vi "Simple Client - Front Panel.vi"() -> ()   [LabVIEW 2011]
uses:
  <vilib>/variable/tagger/epics/API/internal/List Records (By Ref).vi
  <vilib>/variable/tagger/epics/API/NI_EPICS_Client.lvlib
  <vilib>/lvdsc/NI_DSC.lvlib
  Program Files (x86)/National Instruments/LabVIEW 2011/resource/objmgr/nvio.rc
panel:
  in  "Host":string="localhost" caption="IOC Host"
  in  "Process Variable":string caption="Process Variable to Read (Numeric Only)"
  in  "Exit":bool
  out "Value History":dbl(graph)
  out "Value":dbl(knob) scale=-100.0..100.0
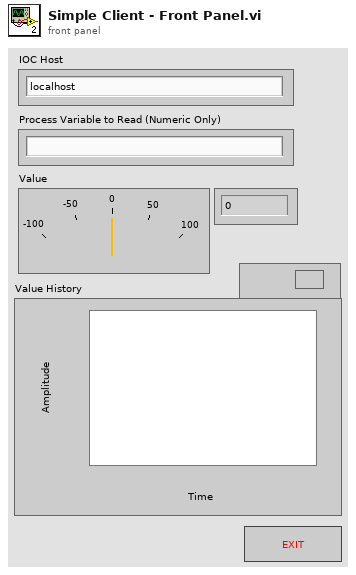
[diagram p1: front panel]
types:
  T1 = enum32{"u32BitField", "bool", "double", "string", "int8", "uint8", "int16", "uint16", "int32", "uint32", "int64", "uint64", "single", "double waveform", "int16 waveform", "array of boolean", "array of int8", "array of uint8", "array of int16", "array of uint16", "array of int32", "array of uint32", "array of int64", "array of uint64", "array of single", "array of double", "array of double waveform", "array of int16 waveform", "array of string", "variant", "timestamp", "fixed point", "custom"}
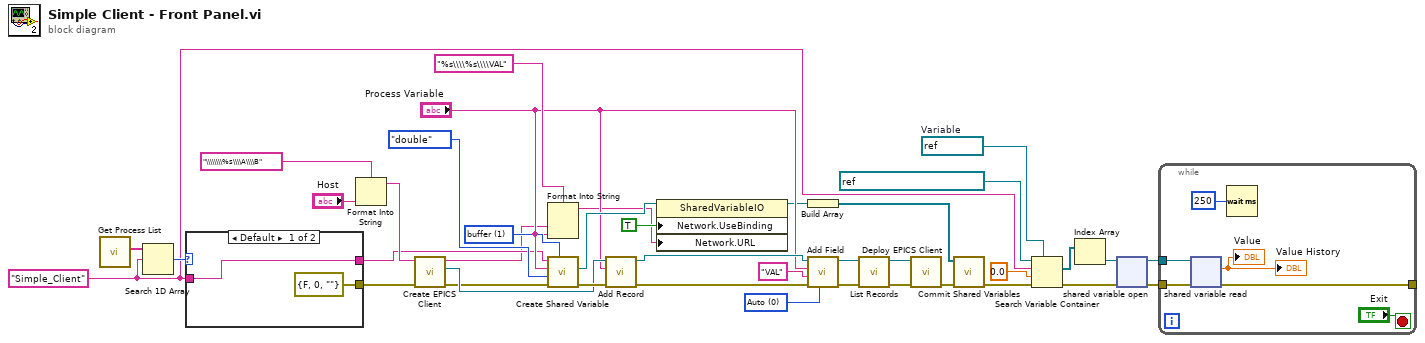
[diagram p0: block diagram]
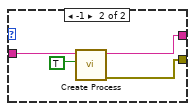
[diagram p2: hidden frame]
diagram:
  w39 = u16 1 items=["commit", "buffer"] ("set mode")
  w24 = refnum<k21> refnum  # Variable
  w2 = "Simple_Client" ("process name")
  w17 = u16 0 items=["Auto", "Double", "Bool", "String", "Short", "Float", "Enum", "Long", "Array of Double"] ("data type")
  n1 = call <vilib>:"Get Process List.vi"() -> ("processes"=w6:string[])  [unwired: 10 in, 1 out]
  n2 = Search 1D Array(1D array=w6, element=w2) -> (index of element=w5:i32)  [unwired: 1 in]
  n3 = case shown="Default" w5 {
    tunnel: [w41 w44] -> w4
    tunnel: [errorcluster {"status"=FALSE, "code"=0, "source"=""} ("error out") w43] -> w3
    tunnel: w2 -> [w41 w42]
    frame Default {
    }
    frame -1 {
      n4 = call <vilib>:"Create Process.vi"("run?"=TRUE, "process name"=w42) -> ("error out"=w43:errorcluster, "process name out"=w44:string)  [unwired: 8 in]
    }
  }
  n5 = Format Into String(format string="\\\\\\\\%s\\\\A\\\\B" ("EPICS Client URL in"), "Host") -> (resulting string=w14:string)  [unwired: 2 in, 1 out]
  n6 = call <vilib>:"Create EPICS Client.vi"("error in (no error)"=w3, "EPICS Client URL in"=w14) -> ("error out"=w31:errorcluster, "EPICS Client ref"=w32:refnum<data-value>, "EPICS Client URL out"=w1:string)  [unwired: 7 in]
  n7 = Format Into String(format string="%s\\\\%s\\\\VAL" ("EPICS Client URL in"), w1, "Process Variable") -> (resulting string=w9:string)  [unwired: 2 in, 1 out]
  n8 = call <vilib>:"Create Shared Variable.vi"("set mode"=w39, "error in (no error)"=w31, "data type"=T1."double", "shared variable name"="Process Variable", "process name"=w4) -> ("error out"=w34:errorcluster, "shared variable"=w36:refnum<k21>)  [unwired: 4 in, 1 out]
  n9 = call <vilib>:"Add Record.vi"("error in (no error)"=w34, "record name"="Process Variable", "EPICS Client ref in"=w32) -> ("error out"=w35:errorcluster, "EPICS Client ref out"=w33:refnum<data-value>)  [unwired: 5 in, 2 out]
  n10 = property class="SharedVariableIO"(reference=w36, "Network.UseBinding"=TRUE ("use binding? (F)"), "Network.URL"=w9) -> (reference out=w7:refnum<k21>)  [unwired: 1 in, 1 out]
  n11 = Build Array(w7) -> (w38:refnum<k21>[])
  n12 = call <vilib>:"Add Field.vi"("data type"=w17, "error in (no error)"=w35, "field name"="VAL", "record name"="Process Variable", "EPICS Client ref in"=w33) -> ("error out"=w18:errorcluster, "EPICS Client ref out"=w19:refnum<data-value>)  [unwired: 3 in, 2 out]
  n13 = call-poly <vilib>:"List Records.vi"("error in (no error)"=w18, "EPICS Client ref in"=w19) -> ("error out"=w21:errorcluster, "EPICS Client ref out"=w20:refnum<data-value>)  [unwired: 7 in, 1 out]
  n14 = call <vilib>:"Deploy EPICS Client.vi"("error in (no error)"=w21, "EPICS Client ref in"=w20) -> ("error out"=w8:errorcluster)  [unwired: 8 in, 1 out]
  n15 = call <vilib>:"Commit Shared Variables.vi"("error in (no error)"=w8, "shared variables"=w38) -> ("error out"=w37:errorcluster)  [unwired: 8 in, 1 out]
  n16 = Search Variable Container(7:w24, 8:w37, 9:0.0, 10:w2, 11:refnum<k21> "ni.var.psp://localhost/" ("container refnum in")) -> (0:w29:errorcluster, 2:w26:refnum<k21>[])  [unwired: 1 in, 1 out]
  n17 = Index Array(array=w26) -> (element=w28:refnum<k21>)  [unwired: 1 in]
  n18 = shared-variable-open(w28, w29) -> (w27:refnum<k21>, w30:errorcluster)  [unwired: 1 in]
  n19 = while {
    tunnel: w27 -> [w50]
    tunnel: w30 -> [w49]
    tunnel: [w46] -> _
    stop <- "Exit" stop-if-true
    n20 = shared-variable-read(w50, w49) -> (w46:errorcluster, →"Value" →"Value History":dbl)  [unwired: 2 out]
    n21 = Wait (ms)(milliseconds to wait=u32 250) -> ()  [unwired: 1 out]
  }
